vi "Configure Average.vi"(0 "VISA resource name":refnum<visa-resource-name>, 5 "error in (no error)":errorcluster, 6 "State":bool) -> (14 "VISA resource name out":refnum<visa-resource-name>, 19 "error out":errorcluster)   [LabVIEW 2020, in "Keithley 2100 Series.lvlib"]
doc: "Definition:\nWhen the Min/Max function is enabled, the multimeter takes in a series of readings from the measurements, stores the minimum and maximum readings in the memory, and then calculates the average value of all readings. The number of readings taken since Min/Max operation is enabled is recorded as well. These data are stored in a volatile memory and will be cleared when the meter is turned off, or when the MIN/MAX is turned on, or after a remote interface reset. The meter beeps every time when it captures a new minimum or maximum.\n\nRemote Interface Operation:\nThe following commands show you how to use the Min/Max operation from your PC terminal.\n\nCALCulate:FUNCtion AVERage\nCALCulate:STATe {OFF|ON}\nCALCulate:STATe?\nCALCulate:AVERage:MINimum?\nCALCulate:AVERage:MAXimum?\nCALCulate:AVERage:AVERage?\nCALCulate:AVERage:COUNt?"
uses:
  Keithley 2100 Series.lvlib
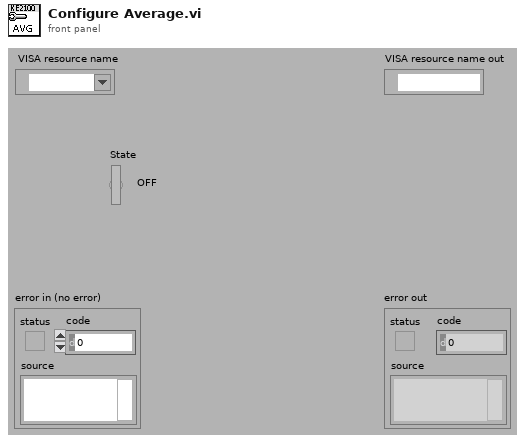
[diagram p1: front panel]
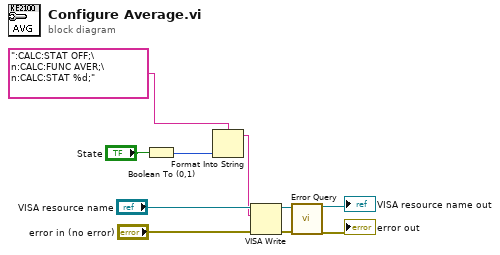
[diagram p0: block diagram]
diagram:
  n1 = Boolean To (0,1)(Boolean="State") -> (0, 1=w3:i16)
  n2 = Format Into String(format string=":CALC:STAT OFF;\n:CALC:FUNC AVER;\n:CALC:STAT %d;", w3) -> (resulting string=w4:string)  [unwired: 2 in, 1 out]
  n3 = VISA Write(VISA resource name="VISA resource name", write buffer=w4, error in (no error)="error in (no error)") -> (VISA resource name out=w9:refnum<visa-resource-name>, error out=w10:errorcluster)  [unwired: 1 out]
  n4 = call "Error Query.vi"("VISA resource name"=w9, "error in (no error)"=w10) -> ("VISA resource name out"=→"VISA resource name out":refnum<visa-resource-name>, "error out"=→"error out":errorcluster)  [unwired: 14 in, 2 out]
